vi "Error Log.vi"() -> ()   [LabVIEW 2016, in "User Interface.lvlib"]
uses:
  User Interface.lvlib
  Error log.ctl
  Create Path Command.ctl
  <vilib>/Utility/file.llb/Write Delimited Spreadsheet (string).vi
panel:
  in  "Command":T1
  in  "Data":string[](array[string])
  out "error out":errorcluster
  in  "error in (no error)":errorcluster
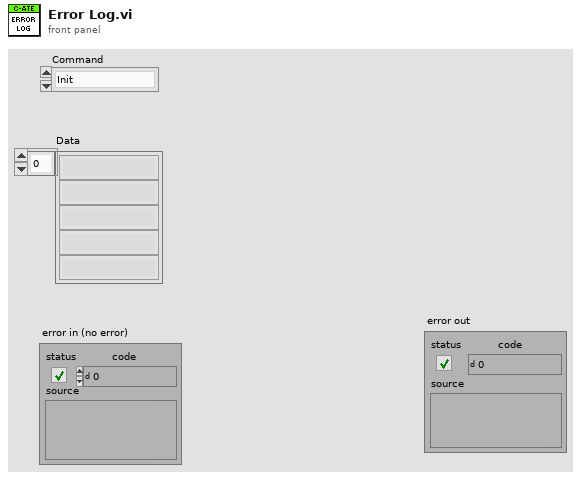
[diagram p1: front panel]
types:
  T1 = typedef "User Interface.lvlib/Error log.ctl" = enum16{"Init", "Read", "Write", "Close"}
  T2 = typedef "User Interface.lvlib/Create Path Command.ctl" = enum16{"Authentication", "Hardware", "Instrument", "Data", "Action log", "Error Log"}
  T3 = enum16{"open", "replace", "create", "open or create", "replace or create", "replace or create with confirmation"}
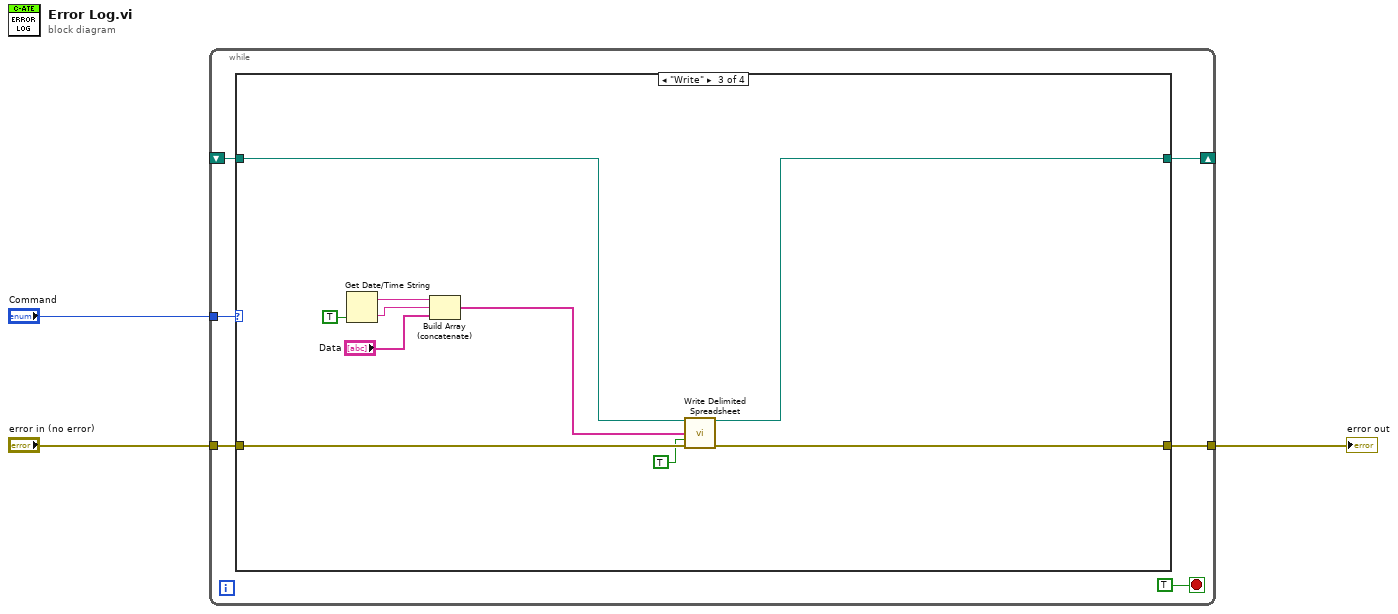
[diagram p0: block diagram]
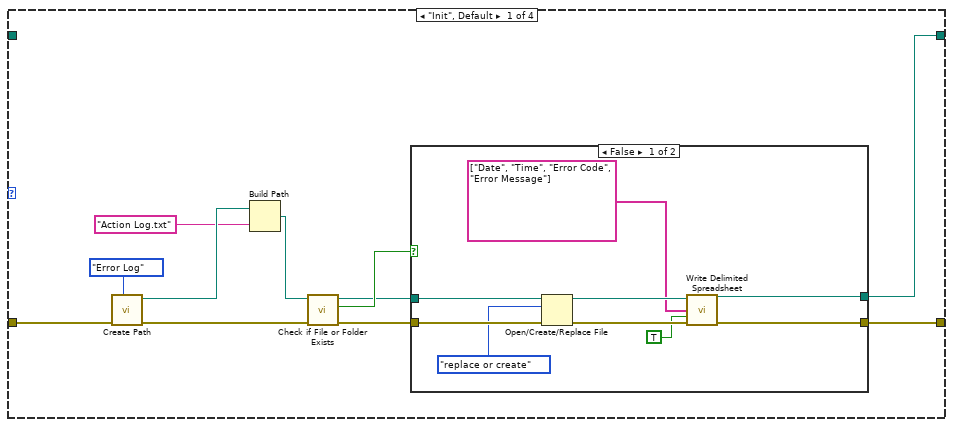
[diagram p2: hidden frame]
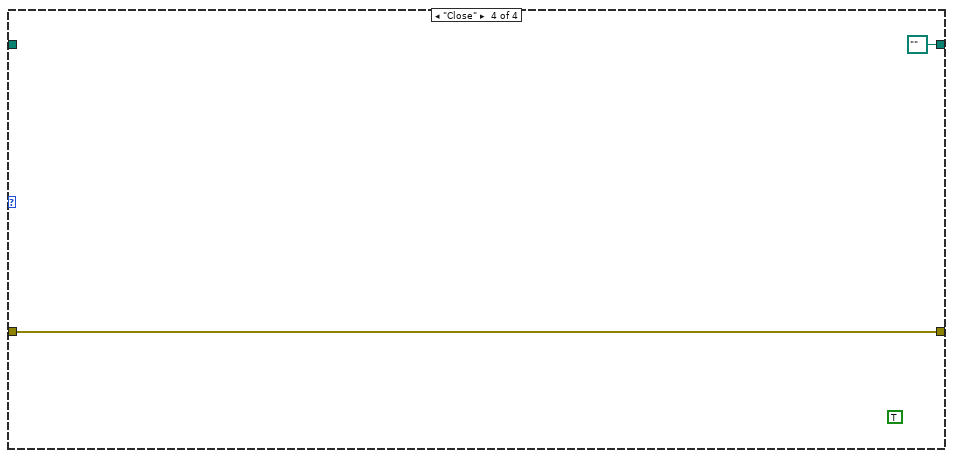
[diagram p5: hidden frame]
diagram:
  n1 = while {
    tunnel: "error in (no error)" -> [w9]
    tunnel: "Command" -> [w8]
    tunnel: [w6] -> w1
    shift-right: [w7] -> _
    shift-left: _ -> [w5]
    stop <- TRUE stop-if-true
    n2 = case shown="\"Write\"" w8 {
      tunnel: w9 -> [w20 _ w40 w41]
      tunnel: [w11 _ w37 path "" ("new file path (Not A Path if cancelled)")] -> w7
      tunnel: [w10 _ w39 w41] -> w6
      tunnel: w5 -> [_ _ w38 _]
      frame "Init", Default {
        n3 = call "Create Path.vi"("Path Command"=Create_Path_Command."Error Log", "error in (no error)"=w20) -> ("error out"=w16:errorcluster, "created path"=w18:path)  [unwired: 8 in]
        n4 = Build Path(base path=w18, name or relative path="Action Log.txt") -> (appended path=w15:path)
        n5 = call <vilib>:"Check if File or Folder Exists.vi"("error in (no error)"=w16, "path"=w15) -> ("error out"=w14:errorcluster, "file or folder exists?"=w13:bool, "dup path"=w12:path)  [unwired: 7 in]
        n6 = case shown="False" w13 {
          tunnel: w14 -> [w28 w29]
          tunnel: w12 -> [w25 w30]
          tunnel: [w23 w29] -> w10
          tunnel: [w22 w30] -> w11
          frame False {
            n7 = Open/Create/Replace File(file path (use dialog)=w25, error in=w28, operation (0:open)=T3."replace or create") -> (error out=w26:errorcluster)  [unwired: 3 in, 2 out]
            n8 = call-poly <vilib>:"Write Delimited Spreadsheet.vi"("file path (dialog if empty)"=w25, "1D data"=string[] ["Date", "Time", "Error Code", "Error Message"], "append to file? (new file:F)"=TRUE, "error in (no error)"=w26) -> ("new file path (Not A Path if cancelled)"=w22:path, "error out"=w23:errorcluster)  [unwired: 10 in]
          }
          frame True {
          }
        }
      }
      frame "Read" {
      }
      frame "Write" {
        n9 = Get Date/Time String(want seconds? (F)=TRUE) -> (date string=w34:string, time string=w33:string)  [unwired: 2 in]
        n10 = Build Array (concatenate)(w34, w33, "Data") -> (w31:string[])
        n11 = call-poly <vilib>:"Write Delimited Spreadsheet.vi"("file path (dialog if empty)"=w38, "1D data"=w31, "append to file? (new file:F)"=TRUE, "error in (no error)"=w40) -> ("new file path (Not A Path if cancelled)"=w37:path, "error out"=w39:errorcluster)  [unwired: 10 in]
      }
      frame "Close" {
        (unwired) TRUE
      }
    }
  }
  "error out" <- w1
